vi "Configure Adapter Rotate.vi"(8 "error in (no error)":errorcluster, 9 "Port (1)":i32=1, 10 "Channel (1)":i32=1, 11 "VISA resource name":refnum<visa-resource-name>) -> (0 "error out":errorcluster, 3 "VISA resource name out":refnum<visa-resource-name>)   [LabVIEW 2022 SP3, in "Agilent ENA Series.lvlib"]
doc: "Configures the adapter rotator.\n\n<B>Note:</B>\nThis VI is only valid for E5061B."
uses:
  <instrlib>/Agilent ENA Series/Agilent ENA Series.lvlib
panel:
  # "Note:\nThis VI is not supported by the E5080A and E5080B."
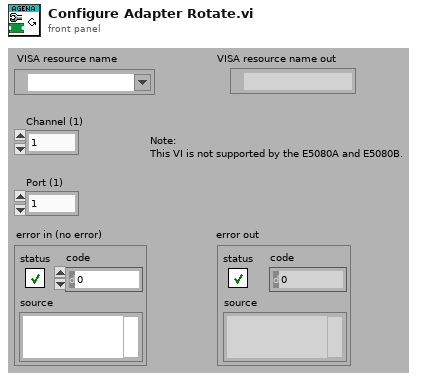
[diagram p1: front panel]
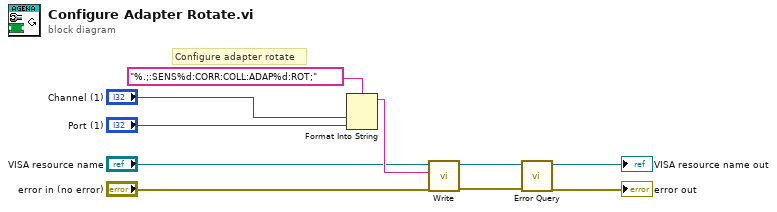
[diagram p0: block diagram]
diagram:
  # "Configure adapter rotate"
  n1 = Format Into String(format string="%.;:SENS%d:CORR:COLL:ADAP%d:ROT;", "Channel (1)", "Port (1)") -> (resulting string=w5:string)  [unwired: 2 in, 1 out]
  n2 = call <instrlib>:"Write.vi"("error in (no error)"="error in (no error)", "String ()"=w5, "VISA resource name"="VISA resource name") -> ("error out"=w1:errorcluster, "VISA resource name out"=w2:refnum<visa-resource-name>)  [unwired: 6 in, 1 out]
  n3 = call <instrlib>:"Error Query.vi"("error in (no error)"=w1, "VISA resource name"=w2) -> ("error out"=→"error out":errorcluster, "VISA resource name out"=→"VISA resource name out":refnum<visa-resource-name>)  [unwired: 8 out]
